vi "Ex10 Fast Fourier Transform.vi"() -> ()   [LabVIEW 2024]
uses:
  <vilib>/vision/NI_Vision_Development_Module.lvlib
panel:
  in  "Operation":u16(ring) items=["Truncate", "Truncate & IFT"]
  in  "Low pass/High pass (Low pass)":bool
  in  "Truncation Frequency %":sgl=10.0 format="%.2f"
  out "error out":errorcluster
  out "Color Channel":T1(plugin-control)
  out "Image":T1(plugin-control)
  in  "Color Plane":i32(ring)=1 items=["Red", "Green", "Blue", "Hue", "Saturation", "Luminance", "Value", "Intensity"]
  in  "File Path":path
  # "EX.10 FAST FOURIER TRANSFORM"
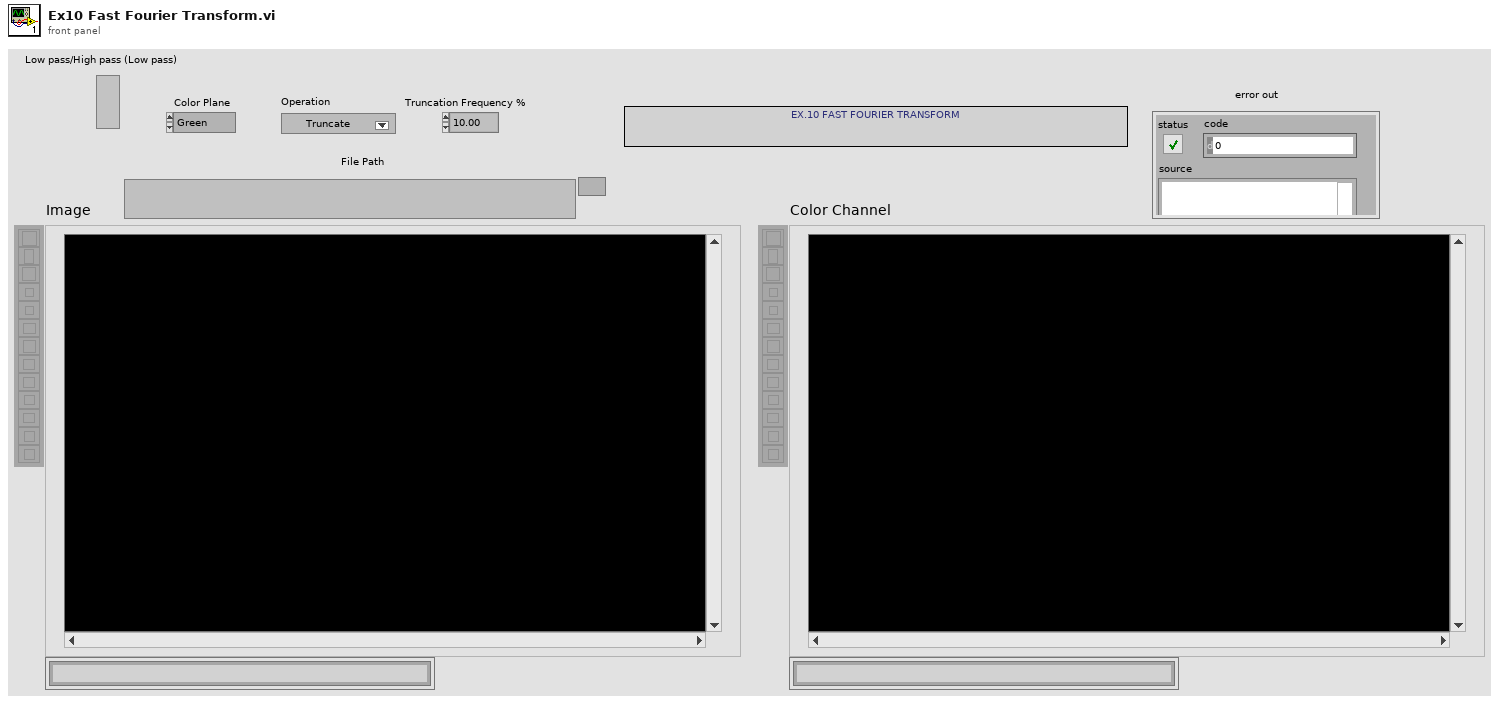
[diagram p1: front panel]
types:
  T1 = typedef "IMAQ Image.ctl" = refnum<image>
  T2 = typedef "Image Type" = u32
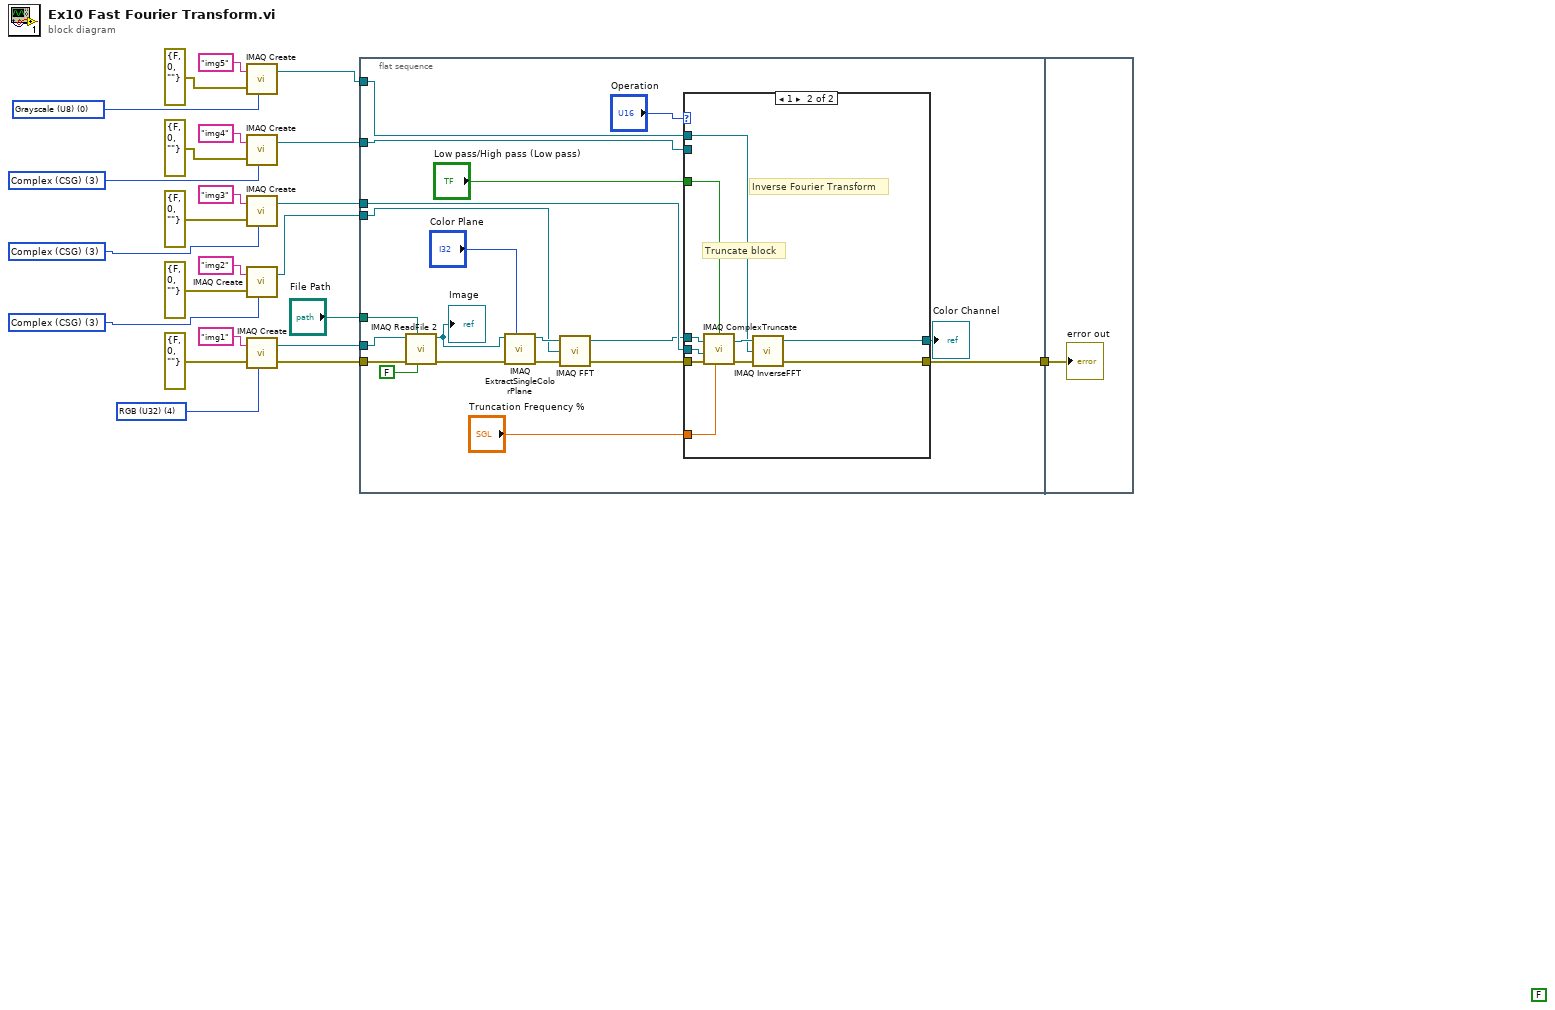
[diagram p0: block diagram]
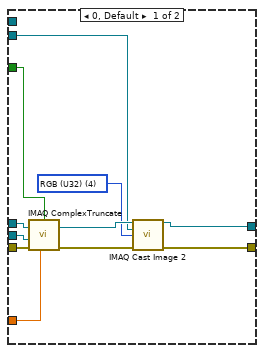
[diagram p2: hidden frame]
diagram:
  w2 = T2 0 items=["Grayscale (U8)", "Grayscale (I16)", "Grayscale (SGL)", "Complex (CSG)", "RGB (U32)", "HSL (U32)", "RGB (U64)", "Grayscale (U16)"] ("Image Type")
  (unwired) FALSE ("status")
  w6 = T2 3 items=["Grayscale (U8)", "Grayscale (I16)", "Grayscale (SGL)", "Complex (CSG)", "RGB (U32)", "HSL (U32)", "RGB (U64)", "Grayscale (U16)"] ("Image Type")
  w10 = T2 3 items=["Grayscale (U8)", "Grayscale (I16)", "Grayscale (SGL)", "Complex (CSG)", "RGB (U32)", "HSL (U32)", "RGB (U64)", "Grayscale (U16)"] ("Image Type")
  w13 = T2 4 items=["Grayscale (U8)", "Grayscale (I16)", "Grayscale (SGL)", "Complex (CSG)", "RGB (U32)", "HSL (U32)", "RGB (U64)", "Grayscale (U16)"] ("Image Type")
  w14 = T2 3 items=["Grayscale (U8)", "Grayscale (I16)", "Grayscale (SGL)", "Complex (CSG)", "RGB (U32)", "HSL (U32)", "RGB (U64)", "Grayscale (U16)"] ("Image Type")
  n1 = call "IMAQ Create"("Image Name"="img5", "Image Type"=w2, "error in (no error)"=errorcluster {"status"=FALSE, "code"=0, "source"=""}) -> ("New Image"=w1:T1)  [unwired: 2 in, 1 out]
  n2 = call "IMAQ Create"("Image Name"="img4", "Image Type"=w6, "error in (no error)"=errorcluster {"status"=FALSE, "code"=0, "source"=""}) -> ("New Image"=w5:T1)  [unwired: 2 in, 1 out]
  n3 = call "IMAQ Create"("Image Name"="img3", "Image Type"=w10, "error in (no error)"=errorcluster {"status"=FALSE, "code"=0, "source"=""}) -> ("New Image"=w9:T1)  [unwired: 2 in, 1 out]
  n4 = call "IMAQ Create"("Image Name"="img2", "Image Type"=w14, "error in (no error)"=errorcluster {"status"=FALSE, "code"=0, "source"=""}) -> ("New Image"=w15:T1)  [unwired: 2 in, 1 out]
  n5 = call "IMAQ Create"("Image Name"="img1", "Image Type"=w13, "error in (no error)"=errorcluster {"status"=FALSE, "code"=0, "source"=""}) -> ("New Image"=w16:T1, "error out"=w17:errorcluster)  [unwired: 2 in]
  n6 = flat-sequence {
    tunnel: "File Path" -> [w42]
    tunnel: w17 -> [w41]
    tunnel: w16 -> [w40]
    tunnel: w15 -> [w34]
    tunnel: [w25] -> w23
    tunnel: w9 -> [w31]
    tunnel: w5 -> [w27]
    tunnel: w1 -> [w24]
    tunnel: w23 -> [w65]
    frame #0 {
      n7 = call "IMAQ ReadFile 2"("Use File Path Image Type"=FALSE, "File Path"=w42, "error in (no error)"=w41, "Image"=w40) -> ("error out"=w38:errorcluster, "Image Out"=w39:T1)  [unwired: 3 in, 3 out]
      "Image" <- w39
      n8 = call "IMAQ ExtractSingleColorPlane"("Color Plane"="Color Plane", "error in (no error)"=w38, "Image Src"=w39) -> ("error out"=w35:errorcluster, "Image Dst Out"=w36:T1)  [unwired: 7 in]
      n9 = call "IMAQ FFT"("error in (no error)"=w35, "Image Dst"=w34, "Image Src"=w36) -> ("error out"=w32:errorcluster, "Image Dst Out"=w29:T1)  [unwired: 1 in]
      n10 = case shown="1" "Operation" {
        tunnel: w32 -> [w54 w63]
        tunnel: w31 -> [w53 w62]
        tunnel: "Truncation Frequency %" -> [w52 w60]
        tunnel: w29 -> [w51 w64]
        tunnel: "Low pass/High pass (Low pass)" -> [w50 w61]
        tunnel: w27 -> [w48 _]
        tunnel: [w47 w56] -> w26
        tunnel: [w46 w55] -> w25
        tunnel: w24 -> [_ w57]
        frame 0, Default {
          w45 = T2 4 items=["Grayscale (U8)", "Grayscale (I16)", "Grayscale (SGL)", "Complex (CSG)", "RGB (U32)", "HSL (U32)", "RGB (U64)", "Grayscale (U16)"] ("Image Type")
          n11 = call "IMAQ ComplexTruncate"("error in (no error)"=w54, "Image Dst"=w53, "Truncation Frequency %"=w52, "Image Src"=w51, "Low pass/High pass (Low pass)"=w50) -> ("error out"=w44:errorcluster, "Image Dst Out"=w49:T1)  [unwired: 2 in]
          n12 = call "IMAQ Cast Image 2"("Image Src"=w49, "Image Dst"=w48, "Image Type"=w45, "error in (no error)"=w44) -> ("Image Dst Out"=w47:T1, "error out"=w46:errorcluster)  [unwired: 10 in]
        }
        frame 1 {
          # "Inverse Fourier Transform"
          # "Truncate block"
          n13 = call "IMAQ ComplexTruncate"("error in (no error)"=w63, "Image Dst"=w62, "Truncation Frequency %"=w60, "Image Src"=w64, "Low pass/High pass (Low pass)"=w61) -> ("error out"=w59:errorcluster, "Image Dst Out"=w58:T1)  [unwired: 2 in]
          n14 = call "IMAQ InverseFFT"("error in (no error)"=w59, "Image Dst"=w57, "Image Src"=w58) -> ("error out"=w55:errorcluster, "Image Dst Out"=w56:T1)  [unwired: 1 in]
        }
      }
      "Color Channel" <- w26
    }
    frame #1 {
      "error out" <- w65
    }
  }
